vi "Tell Reply.vi"(4 "Priority":bool, 6 "Teller":refnum<class "Teller.lvclass">, 7 "Actor in":refnum<class "Actor.lvclass">) -> (0 "Error out":errorcluster)   [LabVIEW 2025, in "_Template.lvlib" / "Templates.lvlib" / "TEMPLATE Msg.lvlib"]
uses:
  TEMPLATE Msg.lvlib
  jettl/jettl/Teller/Teller/Teller.lvclass
  jettl/jettl/Actor/Actor/Actor.lvclass
  TEMPLATE Msg/TEMPLATE Msg.lvclass
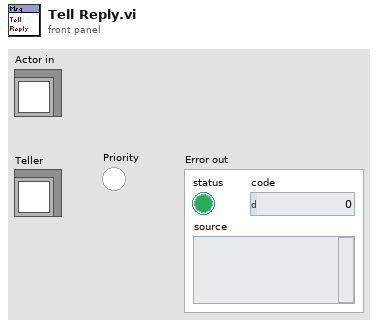
[diagram p1: front panel]
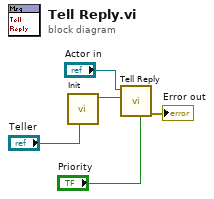
[diagram p0: block diagram]
diagram:
  n1 = call "Init.vi"("Teller"="Teller") -> ("TEMPLATE Msg out"=w2:refnum<class "TEMPLATE Msg.lvclass">)  [unwired: 10 in]
  n2 = call-dynamic "Tell Reply.vi"("Priority"="Priority", "Msg"=w2, "Actor in"="Actor in") -> ("Error out"=→"Error out":errorcluster)  [unwired: 8 in]
